vi "SLSC Control - Battery Switch.vi"() -> ()   [LabVIEW 2014]
doc: "Sample numeric display item."
uses:
  <vilib>/NI Veristand/Display Template Support/Display Template Support.llb/cluster_Screen Item Settings.ctl
  <vilib>/NI Veristand/Display Template Support/Display Template Support.llb/cluster_Graph Scale Settings.ctl
  <vilib>/NI Veristand/Display Template Support/Display Template Support.llb/cluster_Graph Plot Settings.ctl
  Source/Shared/Battery Switch Board/Battery Switch.ctl
  <vilib>/NI Veristand/Display Template Support/Display Template Support.llb/cluster_Graph Handler Message.ctl
  <vilib>/NI Veristand/Display Template Support/Display Template Support.llb/enum_Graph Handler Message.ctl
  <vilib>/NI Veristand/Display Template Support/Display Template Support.llb/sub_Display Template Handler Numeric.vi
  <vilib>/NI Veristand/Display Template Support/Display Template Support.llb/sub_Display Template Data Handler Numeric.vi
  Source/Shared/SLSC configuration Shared.lvlib
panel:
  out "Stop":bool
  in  "Alias":T1
  in  "Item.Data":T2
  in  "Numeric Control":dbl
  out "Label":string="Numeric"
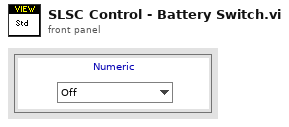
[diagram p1: front panel]
types:
  T1 = typedef "SLSC configuration Shared.lvlib/Battery Switch.ctl" = enum8{"Off", "On"}
  T2 = typedef "cluster_Screen Item Settings.ctl" = cluster{"Template VI":string, "Position X":i32, "Position Y":i32, "Custom":string, "Show Title Bar":bool, "ID":i32, "Always On Top":bool, "Allow Resize":bool, "Allow Minimize":bool, "Allow Close":bool, "Size to Screen":bool, "Screen.ID":i32, "State":enum16{"Normal", "New"}, "Title":string, "Window Bounds":cluster{"[0]":i16, "[1]":i16, "[2]":i16, "[3]":i16}, "Channel Ref":u64, "Unit":string, "Default Units?":bool, "Flash Limit?":bool, "Color 1":u32, "Color 2":u32, "Color 3":u32, "Color 4":u32, "Bck Color":u32, "Fore Color":u32, "Limit 1":dbl, "Limit 2":dbl, "Limit 3":dbl, "Limit 4":dbl, "Limit Mode 1":i32, "Limit Mode 2":i32, "Limit Mode 3":i32, "Limit Mode 4":i32, "Scale Precision":i32, "Scale Min":dbl, "Scale Max":dbl, "Format":i32, "Precision":i32, "Background Type":i32, "IDs":i32[], "Units":string[], "Labels":string[], "Scale Factor":dbl, "Scale Offset":dbl, "YScale Index":u32[], "XScale":T3, "YScales":T3[], "Plots":T4[], "Update Period":dbl, "History Length":dbl, "My.Ref":refnum<vi>, "Is Control?":bool, "Channel Paths":string[], "Custom Data":variant}
  T3 = typedef "cluster_Graph Scale Settings.ctl" = cluster{"Format":u8, "Precision":u8, "Fit":u8, "Label":string, "Use Default Label":bool, "Label Visible":bool, "Min":dbl, "Max":dbl}
  T4 = typedef "cluster_Graph Plot Settings.ctl" = cluster{"Bar Style":u8, "Fill To":i16, "Fill/PtColor":u32, "Line Style":u8, "Line Width":u8, "Color":u32, "Interp":u8, "Point Style":u8}
  T5 = typedef "cluster_Graph Handler Message.ctl" = cluster{"Message":T6, "Data":variant}
  T6 = typedef "enum_Graph Handler Message.ctl" = enum16{"None", "Stop", "Hold", "Update Channels", "New Settings", "Control Value", "Edit Value"}
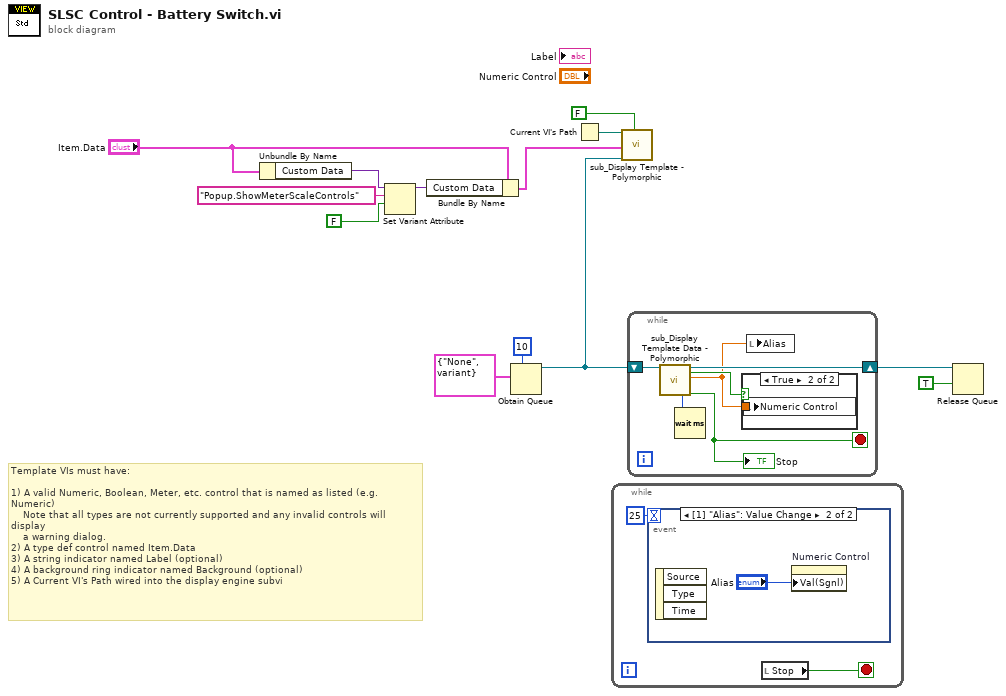
[diagram p0: block diagram]
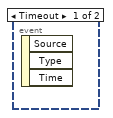
[diagram p2: hidden frame]
diagram:
  # "Template VIs must have:\n\n1) A valid Numeric, Boolean, Meter, etc. control that is named as listed (e.g. Numeric)\n    Note that all types are not currently supported and any invalid controls will display\n    a warning dialog.\n2) A type def control named Item.Data\n3) A string indicator named Label (optional)\n4) A background ring indicator named Background (optional)\n5) A Current VI's Path wired into the display engine subvi"
  n1 = Unbundle By Name("Item.Data") -> ("Custom Data"=w1:variant)
  n2 = Set Variant Attribute(Variant=w1, name="Popup.ShowMeterScaleControls", value=FALSE) -> (Variant out=w4:variant)  [unwired: 1 in, 2 out]
  n3 = Bundle By Name(cluster="Item.Data", "Custom Data"=w4) -> (w6:T2)
  n4 = Obtain Queue(max queue size (-1, unlimited)=10, element data type=T5 {"Message"=enum."None", "Data"=variant} ("Message")) -> (queue out=w8:refnum<queue>)  [unwired: 2 in, 3 out]
  n5 = Current VI's Path() -> (path=w13:path)
  n6 = while {
    stop <- w15 stop-if-true
    n7 = event shown="[1] \"Alias\": Value Change" {
      selector: _ -> [_ _]
      dyn-events: _ -> [_ _]
      timeout: 25 -> [_ _]
      event Timeout {
        n8 = event-data() -> ()  [unwired: 1 in, 3 out]
      }
      event Value Change {
        n9 = event-data() -> ()  [unwired: 1 in, 3 out]
        n10 = property on="Numeric Control" class="DigNum (strict)"("Val(Sgnl)"="Alias") -> ()  [unwired: 2 in, 2 out]
      }
    }
    n11 = local read "Stop"() -> (w15:bool)
  }
  n12 = call-poly <vilib>:"sub_Display Template - Polymorphic.vi"("Parent.Path"=w13, "Item.Data"=w6, "queue"=w8, "Use Transparency?"=FALSE) -> ()  [unwired: 16 out]
  n13 = while {
    shift-right: [w22] -> w12
    shift-left: w8 -> [w21]
    stop <- w19 stop-if-true
    n14 = call-poly <vilib>:"sub_Display Template Data - Polymorphic.vi"("queue"=w21) -> ("Wait.Time"=w20:u32, "queue out"=w22:refnum<queue>, "Update.Value"=w18:bool, "Numeric.Value"=w17:dbl, "Stop"=w19:bool)  [unwired: 14 out]
    "Stop" <- w19
    n15 = Wait (ms)(milliseconds to wait=w20) -> ()  [unwired: 1 out]
    n16 = case shown="True" w18 {
      tunnel: w17 -> [_ w23]
      frame False {
      }
      frame True {
        n17 = local write "Numeric Control"(w23) -> ()
      }
    }
    n18 = local write "Alias"(w17) -> ()
  }
  n19 = Release Queue(queue=w12, force destroy? (F)=TRUE) -> ()  [unwired: 1 in, 3 out]
